vi "5.3 Deg2Fah.vi"() -> ()   [LabVIEW 2019]
uses:
  <vilib>/DAQmx/read.llb/DAQmx Read (Analog DBL 1Chan 1Samp).vi
  <vilib>/DAQmx/miscellaneous.llb/DAQmx Fill In Error Info.vi
panel:
  in  "Scale":bool
  out "Temperature":dbl format="%#_4g"
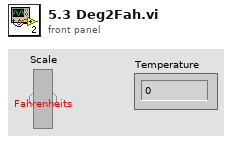
[diagram p1: front panel]
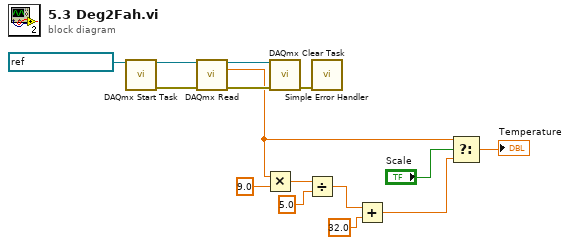
[diagram p0: block diagram]
diagram:
  n1 = call <vilib>:"DAQmx Start Task.vi"("task/channels in"=refnum<k21> "Thermocouple" ("DAQmx Task Name")) -> ("task out"=w14:refnum<k21>, "error out"=w13:errorcluster)  [unwired: 13 in]
  n2 = call-poly <vilib>:"DAQmx Read.vi"("task/channels in"=w14, "error in"=w13) -> ("task out"=w11:refnum<k21>, "data"=w2:dbl, "error out"=w12:errorcluster)  [unwired: 11 in]
  n3 = Multiply(x=w2, y=9.0) -> (x*y=w8:dbl)
  n4 = call <vilib>:"DAQmx Clear Task.vi"("task in"=w11, "error in"=w12) -> ("error out"=w10:errorcluster)  [unwired: 13 in]
  n5 = Divide(x=w8, y=5.0) -> (x/y=w6:dbl)
  n6 = call <vilib>:"Simple Error Handler.vi"("error in (no error)"=w10) -> ()  [unwired: 4 in, 5 out]
  n7 = Add(x=w6, y=32.0) -> (x+y=w4:dbl)
  n8 = Select(t=w2, s="Scale", f=w4) -> (s? t:f=→"Temperature":dbl)
